vi "getSciScan image reference.vi"(8 "Error In":errorcluster, 11 "Image Refnum (Generic)":refnum<vi>) -> (0 "Error Out":errorcluster, 1 "Channel Number":u32, 2 "SciScan Image Tab Number":u32, 3 "Current Image":T1, 4 "Channel type":string)   [LabVIEW 2012]
doc: "SciScan 1.2 160622\nThis SubVI is part of the position control module.\nIts functionality is to manage the UI components related to display of images (in both the top level GUI and the position save UI)"
uses:
  <vilib>/vision/Image Controls.llb/IMAQ Image.ctl
  Custom Controls/display palette control.ctl
  GFG/GFGImageRefsGet.vi
  GFG/GFGfpRefGet.vi
  GFG/GFG library.lvlib
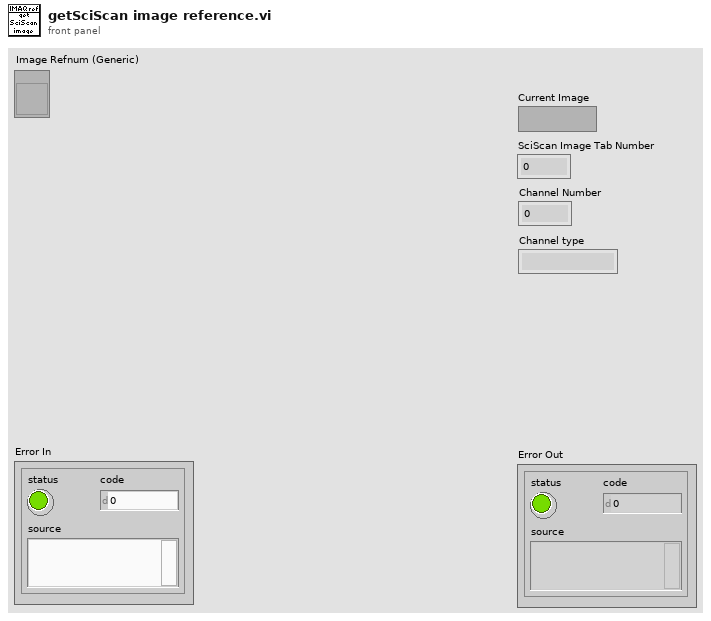
[diagram p1: front panel]
types:
  T1 = typedef "IMAQ Image.ctl" = refnum<image>
  T2 = typedef "display palette control.ctl" = enum16{"standard", "high clipping red", "low clipping blue", "high and low clipping", "high / low (full range)"}
  T3 = cluster{"Channel 1 small":T1, "Channel 2 small":T1, "Channel 3 small":T1, "Channel 4 small":T1, "Channel 1 large":T1, "Channel 2 large":T1, "Channel 3 large":T1, "Channel 4 large":T1, "RGB overlay":T1, "ROI Image display":T1, "arb line scan display":T1, "Channel 5 large":T1}
  T4 = cluster{"WaveformChartRef":refnum<vi>, "DigitalRef":refnum<vi>, "ArrayRef":refnum<vi>, "TabControlRef":refnum<vi>, "EnumRef":refnum<vi>, "RingRef":refnum<vi>, "BooleanRef":refnum<vi>, "KnobRef":refnum<vi>, "SlideRef":refnum<vi>, "PathRef":refnum<vi>, "StringRef":refnum<vi>, "ComboBox":refnum<vi>, "WaveformGraphRef":refnum<vi>}
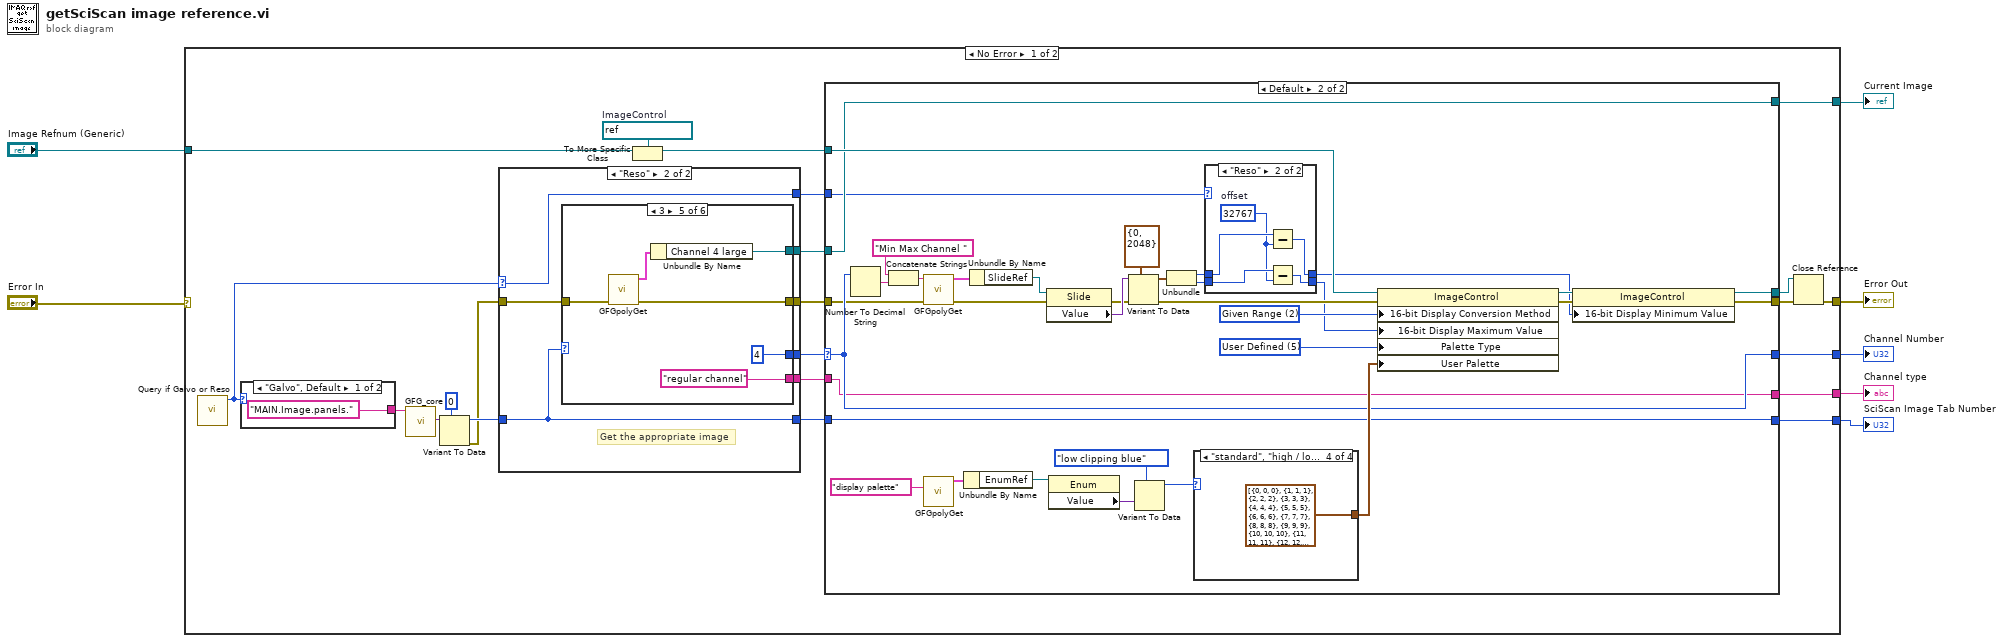
[diagram p0: block diagram]
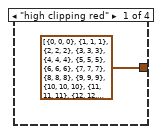
[diagram p4: hidden frame]
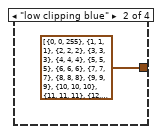
[diagram p5: hidden frame]
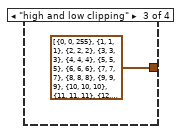
[diagram p6: hidden frame]
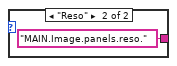
[diagram p7: hidden frame]
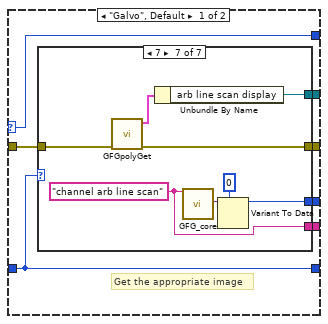
[diagram p8: hidden frame]
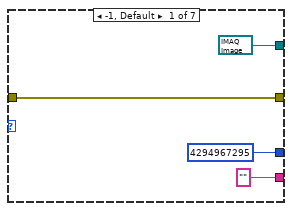
[diagram p9: hidden frame]
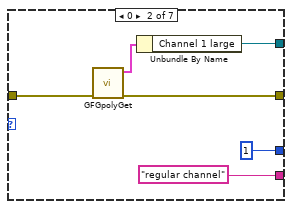
[diagram p10: hidden frame]
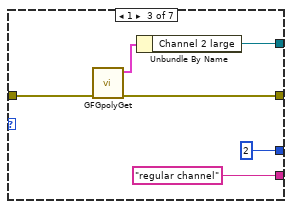
[diagram p11: hidden frame]
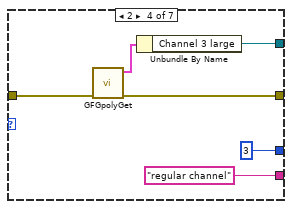
[diagram p12: hidden frame]
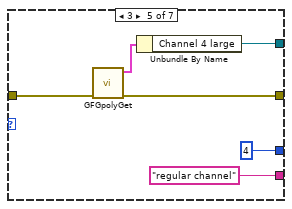
[diagram p13: hidden frame]
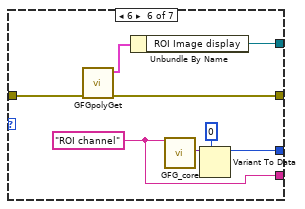
[diagram p14: hidden frame]
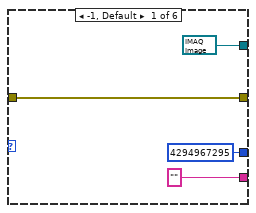
[diagram p15: hidden frame]
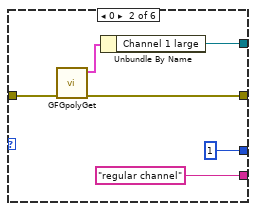
[diagram p16: hidden frame]
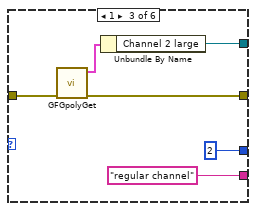
[diagram p17: hidden frame]
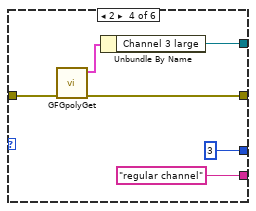
[diagram p18: hidden frame]
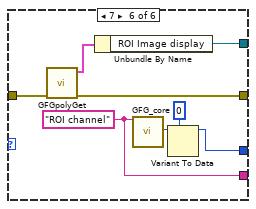
[diagram p19: hidden frame]
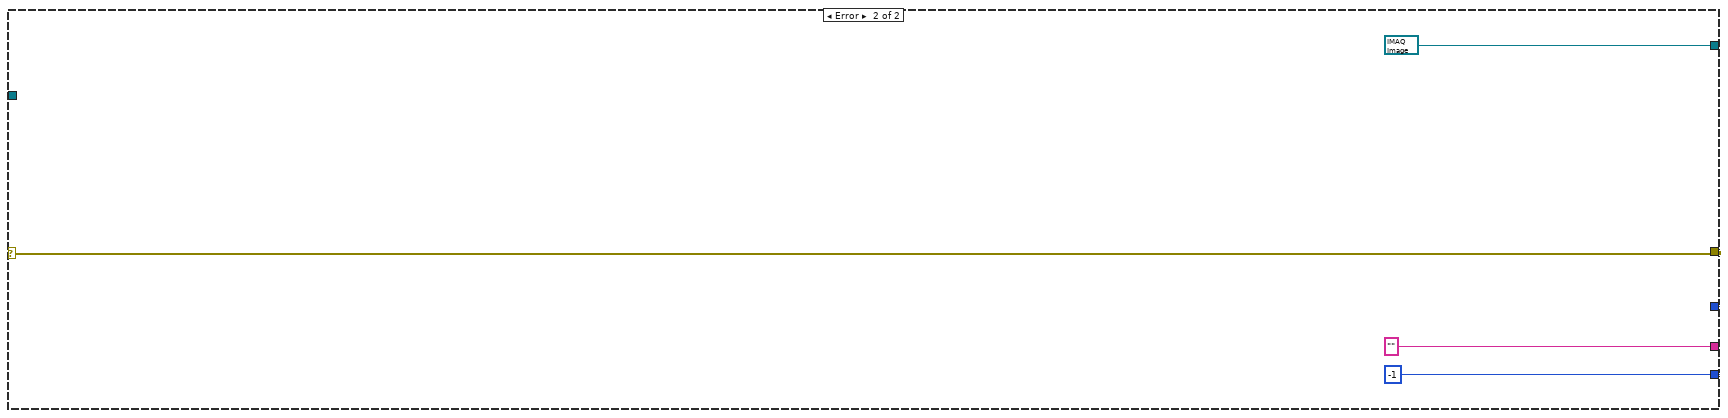
[diagram p20: hidden frame]
diagram:
  n1 = case shown="No Error" "Error In" {
    selector: "Error In" -> [_ w181]
    tunnel: "Image Refnum (Generic)" -> [w17 _]
    tunnel: [w22 w181] -> w5
    tunnel: [w14 T1 refnum ("Channel 4 large")] -> w4
    tunnel: [w11 w179] -> w3
    tunnel: [w13 w179] -> w2
    tunnel: [w9 "" ("Variable Name in")] -> w1
    frame No Error {
      w18 = refnum<vi> refnum  # ImageControl
      n2 = call "Query if Galvo or Reso.vi"() -> ("System Type"=w24:enum16{"Galvo", "Reso"})  [unwired: 10 in, 1 out]
      n3 = case shown="\"Galvo\", Default" w24 {
        tunnel: ["MAIN.Image.panels." ("Variable Name in") "MAIN.Image.panels.reso." ("Variable Name in")] -> w27
        frame "Galvo", Default {
        }
        frame "Reso" {
        }
      }
      n4 = call "GFG_core.vi"("Variable Name in"=w27) -> ("Variant Out"=w25:variant)  [unwired: 12 in, 6 out]
      n5 = Variant To Data(type=u32 0, Variant=w25) -> (data=w23:u32, error out=w21:errorcluster)  [unwired: 1 in]
      n6 = case shown="\"Reso\"" w24 {
        selector: w24 -> [w84 w135]
        tunnel: w21 -> [w90 w141]
        tunnel: w23 -> [w87 w138]
        tunnel: [w89 w140] -> w19
        tunnel: [w88 w139] -> w15
        tunnel: [w87 w138] -> w12
        tunnel: [w86 w137] -> w20
        tunnel: [w85 w136] -> w10
        tunnel: [w84 w135] -> w8
        frame "Galvo", Default {
          # "Get the appropriate image"
          n7 = case shown="7" w87 {
            tunnel: w90 -> [w93 w99 w105 w111 w117 w125 w133]
            tunnel: [w93 w98 w104 w110 w116 w124 w132] -> w89
            tunnel: [T1 refnum ("Channel 4 large") w97 w103 w109 w115 w123 w131] -> w88
            tunnel: [u32 4294967295 u32 1 u32 2 u32 3 u32 4 w120 w128] -> w86
            tunnel: ["" ("Variable Name in") "regular channel" ("Variable Name in") "regular channel" ("Variable Name in") "regular channel" ("Variable Name in") "regular channel" ("Variable Name in") w119 w127] -> w85
            frame -1, Default {
            }
            frame 0 {
              n8 = call-poly "GFGpolyGet.vi"("error in (no error)"=w99) -> ("error out"=w98:errorcluster, "Image Refs Out"=w100:T3)  [unwired: 9 in]
              n9 = Unbundle By Name(w100) -> ("Channel 1 large"=w97:T1)
            }
            frame 1 {
              n10 = call-poly "GFGpolyGet.vi"("error in (no error)"=w105) -> ("error out"=w104:errorcluster, "Image Refs Out"=w106:T3)  [unwired: 9 in]
              n11 = Unbundle By Name(w106) -> ("Channel 2 large"=w103:T1)
            }
            frame 2 {
              n12 = call-poly "GFGpolyGet.vi"("error in (no error)"=w111) -> ("error out"=w110:errorcluster, "Image Refs Out"=w112:T3)  [unwired: 9 in]
              n13 = Unbundle By Name(w112) -> ("Channel 3 large"=w109:T1)
            }
            frame 3 {
              n14 = call-poly "GFGpolyGet.vi"("error in (no error)"=w117) -> ("error out"=w116:errorcluster, "Image Refs Out"=w118:T3)  [unwired: 9 in]
              n15 = Unbundle By Name(w118) -> ("Channel 4 large"=w115:T1)
            }
            frame 6 {
              w119 = "ROI channel" ("Variable Name in")
              n16 = call-poly "GFGpolyGet.vi"("error in (no error)"=w125) -> ("error out"=w124:errorcluster, "Image Refs Out"=w126:T3)  [unwired: 9 in]
              n17 = Unbundle By Name(w126) -> ("ROI Image display"=w123:T1)
              n18 = call "GFG_core.vi"("Variable Name in"=w119) -> ("Variant Out"=w121:variant)  [unwired: 12 in, 6 out]
              n19 = Variant To Data(type=u32 0, Variant=w121) -> (data=w120:u32)  [unwired: 1 in, 1 out]
            }
            frame 7 {
              w127 = "channel arb line scan" ("Variable Name in")
              n20 = call-poly "GFGpolyGet.vi"("error in (no error)"=w133) -> ("error out"=w132:errorcluster, "Image Refs Out"=w134:T3)  [unwired: 9 in]
              n21 = Unbundle By Name(w134) -> ("arb line scan display"=w131:T1)
              n22 = call "GFG_core.vi"("Variable Name in"=w127) -> ("Variant Out"=w129:variant)  [unwired: 12 in, 6 out]
              n23 = Variant To Data(type=u32 0, Variant=w129) -> (data=w128:u32)  [unwired: 1 in, 1 out]
            }
          }
        }
        frame "Reso" {
          # "Get the appropriate image"
          n24 = case shown="3" w138 {
            tunnel: w141 -> [w144 w150 w156 w162 w168 w176]
            tunnel: [w144 w149 w155 w161 w167 w175] -> w140
            tunnel: [T1 refnum ("Channel 4 large") w148 w154 w160 w166 w174] -> w139
            tunnel: [u32 4294967295 u32 1 u32 2 u32 3 u32 4 w171] -> w137
            tunnel: ["" ("Variable Name in") "regular channel" ("Variable Name in") "regular channel" ("Variable Name in") "regular channel" ("Variable Name in") "regular channel" ("Variable Name in") w170] -> w136
            frame -1, Default {
            }
            frame 0 {
              n25 = call-poly "GFGpolyGet.vi"("error in (no error)"=w150) -> ("error out"=w149:errorcluster, "Image Refs Out"=w151:T3)  [unwired: 9 in]
              n26 = Unbundle By Name(w151) -> ("Channel 1 large"=w148:T1)
            }
            frame 1 {
              n27 = call-poly "GFGpolyGet.vi"("error in (no error)"=w156) -> ("error out"=w155:errorcluster, "Image Refs Out"=w157:T3)  [unwired: 9 in]
              n28 = Unbundle By Name(w157) -> ("Channel 2 large"=w154:T1)
            }
            frame 2 {
              n29 = call-poly "GFGpolyGet.vi"("error in (no error)"=w162) -> ("error out"=w161:errorcluster, "Image Refs Out"=w163:T3)  [unwired: 9 in]
              n30 = Unbundle By Name(w163) -> ("Channel 3 large"=w160:T1)
            }
            frame 3 {
              n31 = call-poly "GFGpolyGet.vi"("error in (no error)"=w168) -> ("error out"=w167:errorcluster, "Image Refs Out"=w169:T3)  [unwired: 9 in]
              n32 = Unbundle By Name(w169) -> ("Channel 4 large"=w166:T1)
            }
            frame 7 {
              w170 = "ROI channel" ("Variable Name in")
              n33 = call-poly "GFGpolyGet.vi"("error in (no error)"=w176) -> ("error out"=w175:errorcluster, "Image Refs Out"=w177:T3)  [unwired: 9 in]
              n34 = Unbundle By Name(w177) -> ("ROI Image display"=w174:T1)
              n35 = call "GFG_core.vi"("Variable Name in"=w170) -> ("Variant Out"=w172:variant)  [unwired: 12 in, 6 out]
              n36 = Variant To Data(type=u32 0, Variant=w172) -> (data=w171:u32)  [unwired: 1 in, 1 out]
            }
          }
        }
      }
      n37 = To More Specific Class(target class=w18, reference=w17) -> (specific class reference=w16:refnum<vi>)  [unwired: 1 in, 1 out]
      n38 = case shown="Default" w20 {
        selector: w20 -> [w32 w44]
        tunnel: w16 -> [w35 w46]
        tunnel: [w35 w48] -> w29
        tunnel: [w34 w47] -> w28
        tunnel: w19 -> [w34 w41]
        tunnel: w15 -> [w33 w45]
        tunnel: [w33 w45] -> w14
        tunnel: [w32 w44] -> w13
        tunnel: w12 -> [w31 w43]
        tunnel: [w31 w43] -> w11
        tunnel: w10 -> [w30 w42]
        tunnel: [w30 w42] -> w9
        tunnel: w8 -> [_ w40]
        frame 0, -1 {
        }
        frame Default {
          w52 = u32 5 items=["Grayscale", "Binary", "Gradient", "Rainbow", "Temperature", "User Defined"] ("Palette:Palette Type")
          w63 = u32 2 items=["Full Dynamic", "Downshift", "Given Range", "90% Dynamic", "Given Percent Range"] ("16-bit Display Mapping:Conversion Method")
          n39 = Number To Decimal String(number=w44) -> (decimal integer string=w66:string)  [unwired: 1 in]
          n40 = Concatenate Strings("Min Max Channel " ("Variable Name in"), w66) -> (w70:string)
          n41 = call-poly "GFGpolyGet.vi"("error in (no error)"=w41, "Variable Name in"=w70) -> ("error out"=w62:errorcluster, "output cluster"=w64:T4)  [unwired: 8 in]
          n42 = call-poly "GFGpolyGet.vi"("Variable Name in"="display palette") -> ("output cluster"=w56:T4)  [unwired: 9 in, 1 out]
          n43 = Unbundle By Name(w56) -> ("EnumRef"=w57:refnum<vi>)
          n44 = Unbundle By Name(w64) -> ("SlideRef"=w67:refnum<vi>)
          n45 = property class="Slide"(reference=w67, error in=w62) -> (error out=w61:errorcluster, "Value"=w68:variant)  [unwired: 1 out]
          n46 = property class="Enum"(reference=w57) -> ("Value"=w55:variant)  [unwired: 1 in, 2 out]
          n47 = Variant To Data(error in=w61, type=cluster{i32, i32} {0, 2048} ("channel1"), Variant=w68) -> (data=w59:cluster{i32, i32}, error out=w60:errorcluster)
          n48 = Variant To Data(type=display_palette_control."low clipping blue" ("display palette"), Variant=w55) -> (data=w53:T2)  [unwired: 1 in, 1 out]
          n49 = Unbundle(w59) -> (w39:i32, w38:i32)
          n50 = case shown="\"standard\", \"high / low (full range)\"" w53 {
            tunnel: [cluster{"Red":u8, "Green":u8, "Blue":u8}[] [{"Red"=0, "Green"=0, "Blue"=0}, {"Red"=1, "Green"=1, "Blue"=1}, {"Red"=2, "Green"=2, "Blue"=2}, {"Red"=3, "Green"=3, "Blue"=3}, {"Red"=4, "Green"=4, "Blue"=4}, {"Red"=5, "Green"=5, "Blue"=5}, {"Red"=6, "Green"=6, "Blue"=6}, {"Red"=7, "Green"=7, "Blue"=7}, {"Red"=8, "Green"=8, "Blue"=8}, {"Red"=9, "Green"=9, "Blue"=9}, {"Red"=10, "Green"=10, "Blue"=10}, {"Red"=11, "Green"=11, "Blue"=11}, {"Red"=12, "Green"=12, "Blue"=12}, {"Red"=13, "Green"=13, "Blue"=13}, {"Red"=14, "Green"=14, "Blue"=14}, {"Red"=15, "Green"=15, "Blue"=15}, {"Red"=16, "Green"=16, "Blue"=16}, {"Red"=17, "Green"=17, "Blue"=17}, {"Red"=18, "Green"=18, "Blue"=18}, {"Red"=19, "Green"=19, "Blue"=19}, {"Red"=20, "Green"=20, "Blue"=20}, {"Red"=21, "Green"=21, "Blue"=21}, {"Red"=22, "Green"=22, "Blue"=22}, {"Red"=23, "Green"=23, "Blue"=23}, {"Red"=24, "Green"=24, "Blue"=24}, {"Red"=25, "Green"=25, "Blue"=25}, {"Red"=26, "Green"=26, "Blue"=26}, {"Red"=27, "Green"=27, "Blue"=27}, {"Red"=28, "Green"=28, "Blue"=28}, {"Red"=29, "Green"=29, "Blue"=29}, {"Red"=30, "Green"=30, "Blue"=30}, {"Red"=31, "Green"=31, "Blue"=31}, {"Red"=32, "Green"=32, "Blue"=32}, {"Red"=33, "Green"=33, "Blue"=33}, {"Red"=34, "Green"=34, "Blue"=34}, {"Red"=35, "Green"=35, "Blue"=35}, {"Red"=36, "Green"=36, "Blue"=36}, {"Red"=37, "Green"=37, "Blue"=37}, {"Red"=38, "Green"=38, "Blue"=38}, {"Red"=39, "Green"=39, "Blue"=39}, {"Red"=40, "Green"=40, "Blue"=40}, {"Red"=41, "Green"=41, "Blue"=41}, {"Red"=42, "Green"=42, "Blue"=42}, {"Red"=43, "Green"=43, "Blue"=43}, {"Red"=44, "Green"=44, "Blue"=44}, {"Red"=45, "Green"=45, "Blue"=45}, {"Red"=46, "Green"=46, "Blue"=46}, {"Red"=47, "Green"=47, "Blue"=47}, {"Red"=48, "Green"=48, "Blue"=48}, {"Red"=49, "Green"=49, "Blue"=49}, {"Red"=50, "Green"=50, "Blue"=50}, {"Red"=51, "Green"=51, "Blue"=51}, {"Red"=52, "Green"=52, "Blue"=52}, {"Red"=53, "Green"=53, "Blue"=53}, {"Red"=54, "Green"=54, "Blue"=54}, {"Red"=55, "Green"=55, "Blue"=55}, {"Red"=56, "Green"=56, "Blue"=56}, {"Red"=57, "Green"=57, "Blue"=57}, {"Red"=58, "Green"=58, "Blue"=58}, {"Red"=59, "Green"=59, "Blue"=59}, {"Red"=60, "Green"=60, "Blue"=60}, {"Red"=61, "Green"=61, "Blue"=61}, {"Red"=62, "Green"=62, "Blue"=62}, {"Red"=63, "Green"=63, "Blue"=63}, {"Red"=64, "Green"=64, "Blue"=64}, {"Red"=65, "Green"=65, "Blue"=65}, {"Red"=66, "Green"=66, "Blue"=66}, {"Red"=67, "Green"=67, "Blue"=67}, {"Red"=68, "Green"=68, "Blue"=68}, {"Red"=69, "Green"=69, "Blue"=69}, {"Red"=70, "Green"=70, "Blue"=70}, {"Red"=71, "Green"=71, "Blue"=71}, {"Red"=72, "Green"=72, "Blue"=72}, {"Red"=73, "Green"=73, "Blue"=73}, {"Red"=74, "Green"=74, "Blue"=74}, {"Red"=75, "Green"=75, "Blue"=75}, {"Red"=76, "Green"=76, "Blue"=76}, {"Red"=77, "Green"=77, "Blue"=77}, {"Red"=78, "Green"=78, "Blue"=78}, {"Red"=79, "Green"=79, "Blue"=79}, {"Red"=80, "Green"=80, "Blue"=80}, {"Red"=81, "Green"=81, "Blue"=81}, {"Red"=82, "Green"=82, "Blue"=82}, {"Red"=83, "Green"=83, "Blue"=83}, {"Red"=84, "Green"=84, "Blue"=84}, {"Red"=85, "Green"=85, "Blue"=85}, {"Red"=86, "Green"=86, "Blue"=86}, {"Red"=87, "Green"=87, "Blue"=87}, {"Red"=88, "Green"=88, "Blue"=88}, {"Red"=89, "Green"=89, "Blue"=89}, {"Red"=90, "Green"=90, "Blue"=90}, {"Red"=91, "Green"=91, "Blue"=91}, {"Red"=92, "Green"=92, "Blue"=92}, {"Red"=93, "Green"=93, "Blue"=93}, {"Red"=94, "Green"=94, "Blue"=94}, {"Red"=95, "Green"=95, "Blue"=95}, {"Red"=96, "Green"=96, "Blue"=96}, {"Red"=97, "Green"=97, "Blue"=97}, {"Red"=98, "Green"=98, "Blue"=98}, {"Red"=99, "Green"=99, "Blue"=99}, {"Red"=100, "Green"=100, "Blue"=100}, {"Red"=101, "Green"=101, "Blue"=101}, {"Red"=102, "Green"=102, "Blue"=102}, {"Red"=103, "Green"=103, "Blue"=103}, {"Red"=104, "Green"=104, "Blue"=104}, {"Red"=105, "Green"=105, "Blue"=105}, {"Red"=106, "Green"=106, "Blue"=106}, {"Red"=107, "Green"=107, "Blue"=107}, {"Red"=108, "Green"=108, "Blue"=108}, {"Red"=109, "Green"=109, "Blue"=109}, {"Red"=110, "Green"=110, "Blue"=110}, {"Red"=111, "Green"=111, "Blue"=111}, {"Red"=112, "Green"=112, "Blue"=112}, {"Red"=113, "Green"=113, "Blue"=113}, {"Red"=114, "Green"=114, "Blue"=114}, {"Red"=115, "Green"=115, "Blue"=115}, {"Red"=116, "Green"=116, "Blue"=116}, {"Red"=117, "Green"=117, "Blue"=117}, {"Red"=118, "Green"=118, "Blue"=118}, {"Red"=119, "Green"=119, "Blue"=119}, {"Red"=120, "Green"=120, "Blue"=120}, {"Red"=121, "Green"=121, "Blue"=121}, {"Red"=122, "Green"=122, "Blue"=122}, {"Red"=123, "Green"=123, "Blue"=123}, {"Red"=124, "Green"=124, "Blue"=124}, {"Red"=125, "Green"=125, "Blue"=125}, {"Red"=126, "Green"=126, "Blue"=126}, {"Red"=127, "Green"=127, "Blue"=127}, {"Red"=128, "Green"=128, "Blue"=128}, {"Red"=129, "Green"=129, "Blue"=129}, {"Red"=130, "Green"=130, "Blue"=130}, {"Red"=131, "Green"=131, "Blue"=131}, {"Red"=132, "Green"=132, "Blue"=132}, {"Red"=133, "Green"=133, "Blue"=133}, {"Red"=134, "Green"=134, "Blue"=134}, {"Red"=135, "Green"=135, "Blue"=135}, {"Red"=136, "Green"=136, "Blue"=136}, {"Red"=137, "Green"=137, "Blue"=137}, {"Red"=138, "Green"=138, "Blue"=138}, {"Red"=139, "Green"=139, "Blue"=139}, {"Red"=140, "Green"=140, "Blue"=140}, {"Red"=141, "Green"=141, "Blue"=141}, {"Red"=142, "Green"=142, "Blue"=142}, {"Red"=143, "Green"=143, "Blue"=143}, {"Red"=144, "Green"=144, "Blue"=144}, {"Red"=145, "Green"=145, "Blue"=145}, {"Red"=146, "Green"=146, "Blue"=146}, {"Red"=147, "Green"=147, "Blue"=147}, {"Red"=148, "Green"=148, "Blue"=148}, {"Red"=149, "Green"=149, "Blue"=149}, {"Red"=150, "Green"=150, "Blue"=150}, {"Red"=151, "Green"=151, "Blue"=151}, {"Red"=152, "Green"=152, "Blue"=152}, {"Red"=153, "Green"=153, "Blue"=153}, {"Red"=154, "Green"=154, "Blue"=154}, {"Red"=155, "Green"=155, "Blue"=155}, {"Red"=156, "Green"=156, "Blue"=156}, {"Red"=157, "Green"=157, "Blue"=157}, {"Red"=158, "Green"=158, "Blue"=158}, {"Red"=159, "Green"=159, "Blue"=159}, {"Red"=160, "Green"=160, "Blue"=160}, {"Red"=161, "Green"=161, "Blue"=161}, {"Red"=162, "Green"=162, "Blue"=162}, {"Red"=163, "Green"=163, "Blue"=163}, {"Red"=164, "Green"=164, "Blue"=164}, {"Red"=165, "Green"=165, "Blue"=165}, {"Red"=166, "Green"=166, "Blue"=166}, {"Red"=167, "Green"=167, "Blue"=167}, {"Red"=168, "Green"=168, "Blue"=168}, {"Red"=169, "Green"=169, "Blue"=169}, {"Red"=170, "Green"=170, "Blue"=170}, {"Red"=171, "Green"=171, "Blue"=171}, {"Red"=172, "Green"=172, "Blue"=172}, {"Red"=173, "Green"=173, "Blue"=173}, {"Red"=174, "Green"=174, "Blue"=174}, {"Red"=175, "Green"=175, "Blue"=175}, {"Red"=176, "Green"=176, "Blue"=176}, {"Red"=177, "Green"=177, "Blue"=177}, {"Red"=178, "Green"=178, "Blue"=178}, {"Red"=179, "Green"=179, "Blue"=179}, {"Red"=180, "Green"=180, "Blue"=180}, {"Red"=181, "Green"=181, "Blue"=181}, {"Red"=182, "Green"=182, "Blue"=182}, {"Red"=183, "Green"=183, "Blue"=183}, {"Red"=184, "Green"=184, "Blue"=184}, {"Red"=185, "Green"=185, "Blue"=185}, {"Red"=186, "Green"=186, "Blue"=186}, {"Red"=187, "Green"=187, "Blue"=187}, {"Red"=188, "Green"=188, "Blue"=188}, {"Red"=189, "Green"=189, "Blue"=189}, {"Red"=190, "Green"=190, "Blue"=190}, {"Red"=191, "Green"=191, "Blue"=191}, {"Red"=192, "Green"=192, "Blue"=192}, {"Red"=193, "Green"=193, "Blue"=193}, {"Red"=194, "Green"=194, "Blue"=194}, {"Red"=195, "Green"=195, "Blue"=195}, {"Red"=196, "Green"=196, "Blue"=196}, {"Red"=197, "Green"=197, "Blue"=197}, {"Red"=198, "Green"=198, "Blue"=198}, {"Red"=199, "Green"=199, "Blue"=199}, {"Red"=200, "Green"=200, "Blue"=200}, {"Red"=201, "Green"=201, "Blue"=201}, {"Red"=202, "Green"=202, "Blue"=202}, {"Red"=203, "Green"=203, "Blue"=203}, {"Red"=204, "Green"=204, "Blue"=204}, {"Red"=205, "Green"=205, "Blue"=205}, {"Red"=206, "Green"=206, "Blue"=206}, {"Red"=207, "Green"=207, "Blue"=207}, {"Red"=208, "Green"=208, "Blue"=208}, {"Red"=209, "Green"=209, "Blue"=209}, {"Red"=210, "Green"=210, "Blue"=210}, {"Red"=211, "Green"=211, "Blue"=211}, {"Red"=212, "Green"=212, "Blue"=212}, {"Red"=213, "Green"=213, "Blue"=213}, {"Red"=214, "Green"=214, "Blue"=214}, {"Red"=215, "Green"=215, "Blue"=215}, {"Red"=216, "Green"=216, "Blue"=216}, {"Red"=217, "Green"=217, "Blue"=217}, {"Red"=218, "Green"=218, "Blue"=218}, {"Red"=219, "Green"=219, "Blue"=219}, {"Red"=220, "Green"=220, "Blue"=220}, {"Red"=221, "Green"=221, "Blue"=221}, {"Red"=222, "Green"=222, "Blue"=222}, {"Red"=223, "Green"=223, "Blue"=223}, {"Red"=224, "Green"=224, "Blue"=224}, {"Red"=225, "Green"=225, "Blue"=225}, {"Red"=226, "Green"=226, "Blue"=226}, {"Red"=227, "Green"=227, "Blue"=227}, {"Red"=228, "Green"=228, "Blue"=228}, {"Red"=229, "Green"=229, "Blue"=229}, {"Red"=230, "Green"=230, "Blue"=230}, {"Red"=231, "Green"=231, "Blue"=231}, {"Red"=232, "Green"=232, "Blue"=232}, {"Red"=233, "Green"=233, "Blue"=233}, {"Red"=234, "Green"=234, "Blue"=234}, {"Red"=235, "Green"=235, "Blue"=235}, {"Red"=236, "Green"=236, "Blue"=236}, {"Red"=237, "Green"=237, "Blue"=237}, {"Red"=238, "Green"=238, "Blue"=238}, {"Red"=239, "Green"=239, "Blue"=239}, {"Red"=240, "Green"=240, "Blue"=240}, {"Red"=241, "Green"=241, "Blue"=241}, {"Red"=242, "Green"=242, "Blue"=242}, {"Red"=243, "Green"=243, "Blue"=243}, {"Red"=244, "Green"=244, "Blue"=244}, {"Red"=245, "Green"=245, "Blue"=245}, {"Red"=246, "Green"=246, "Blue"=246}, {"Red"=247, "Green"=247, "Blue"=247}, {"Red"=248, "Green"=248, "Blue"=248}, {"Red"=249, "Green"=249, "Blue"=249}, {"Red"=250, "Green"=250, "Blue"=250}, {"Red"=251, "Green"=251, "Blue"=251}, {"Red"=252, "Green"=252, "Blue"=252}, {"Red"=253, "Green"=253, "Blue"=253}, {"Red"=254, "Green"=254, "Blue"=254}, {"Red"=255, "Green"=0, "Blue"=0}] ("Color Palette") cluster{"Red":u8, "Green":u8, "Blue":u8}[] [{"Red"=0, "Green"=0, "Blue"=255}, {"Red"=1, "Green"=1, "Blue"=1}, {"Red"=2, "Green"=2, "Blue"=2}, {"Red"=3, "Green"=3, "Blue"=3}, {"Red"=4, "Green"=4, "Blue"=4}, {"Red"=5, "Green"=5, "Blue"=5}, {"Red"=6, "Green"=6, "Blue"=6}, {"Red"=7, "Green"=7, "Blue"=7}, {"Red"=8, "Green"=8, "Blue"=8}, {"Red"=9, "Green"=9, "Blue"=9}, {"Red"=10, "Green"=10, "Blue"=10}, {"Red"=11, "Green"=11, "Blue"=11}, {"Red"=12, "Green"=12, "Blue"=12}, {"Red"=13, "Green"=13, "Blue"=13}, {"Red"=14, "Green"=14, "Blue"=14}, {"Red"=15, "Green"=15, "Blue"=15}, {"Red"=16, "Green"=16, "Blue"=16}, {"Red"=17, "Green"=17, "Blue"=17}, {"Red"=18, "Green"=18, "Blue"=18}, {"Red"=19, "Green"=19, "Blue"=19}, {"Red"=20, "Green"=20, "Blue"=20}, {"Red"=21, "Green"=21, "Blue"=21}, {"Red"=22, "Green"=22, "Blue"=22}, {"Red"=23, "Green"=23, "Blue"=23}, {"Red"=24, "Green"=24, "Blue"=24}, {"Red"=25, "Green"=25, "Blue"=25}, {"Red"=26, "Green"=26, "Blue"=26}, {"Red"=27, "Green"=27, "Blue"=27}, {"Red"=28, "Green"=28, "Blue"=28}, {"Red"=29, "Green"=29, "Blue"=29}, {"Red"=30, "Green"=30, "Blue"=30}, {"Red"=31, "Green"=31, "Blue"=31}, {"Red"=32, "Green"=32, "Blue"=32}, {"Red"=33, "Green"=33, "Blue"=33}, {"Red"=34, "Green"=34, "Blue"=34}, {"Red"=35, "Green"=35, "Blue"=35}, {"Red"=36, "Green"=36, "Blue"=36}, {"Red"=37, "Green"=37, "Blue"=37}, {"Red"=38, "Green"=38, "Blue"=38}, {"Red"=39, "Green"=39, "Blue"=39}, {"Red"=40, "Green"=40, "Blue"=40}, {"Red"=41, "Green"=41, "Blue"=41}, {"Red"=42, "Green"=42, "Blue"=42}, {"Red"=43, "Green"=43, "Blue"=43}, {"Red"=44, "Green"=44, "Blue"=44}, {"Red"=45, "Green"=45, "Blue"=45}, {"Red"=46, "Green"=46, "Blue"=46}, {"Red"=47, "Green"=47, "Blue"=47}, {"Red"=48, "Green"=48, "Blue"=48}, {"Red"=49, "Green"=49, "Blue"=49}, {"Red"=50, "Green"=50, "Blue"=50}, {"Red"=51, "Green"=51, "Blue"=51}, {"Red"=52, "Green"=52, "Blue"=52}, {"Red"=53, "Green"=53, "Blue"=53}, {"Red"=54, "Green"=54, "Blue"=54}, {"Red"=55, "Green"=55, "Blue"=55}, {"Red"=56, "Green"=56, "Blue"=56}, {"Red"=57, "Green"=57, "Blue"=57}, {"Red"=58, "Green"=58, "Blue"=58}, {"Red"=59, "Green"=59, "Blue"=59}, {"Red"=60, "Green"=60, "Blue"=60}, {"Red"=61, "Green"=61, "Blue"=61}, {"Red"=62, "Green"=62, "Blue"=62}, {"Red"=63, "Green"=63, "Blue"=63}, {"Red"=64, "Green"=64, "Blue"=64}, {"Red"=65, "Green"=65, "Blue"=65}, {"Red"=66, "Green"=66, "Blue"=66}, {"Red"=67, "Green"=67, "Blue"=67}, {"Red"=68, "Green"=68, "Blue"=68}, {"Red"=69, "Green"=69, "Blue"=69}, {"Red"=70, "Green"=70, "Blue"=70}, {"Red"=71, "Green"=71, "Blue"=71}, {"Red"=72, "Green"=72, "Blue"=72}, {"Red"=73, "Green"=73, "Blue"=73}, {"Red"=74, "Green"=74, "Blue"=74}, {"Red"=75, "Green"=75, "Blue"=75}, {"Red"=76, "Green"=76, "Blue"=76}, {"Red"=77, "Green"=77, "Blue"=77}, {"Red"=78, "Green"=78, "Blue"=78}, {"Red"=79, "Green"=79, "Blue"=79}, {"Red"=80, "Green"=80, "Blue"=80}, {"Red"=81, "Green"=81, "Blue"=81}, {"Red"=82, "Green"=82, "Blue"=82}, {"Red"=83, "Green"=83, "Blue"=83}, {"Red"=84, "Green"=84, "Blue"=84}, {"Red"=85, "Green"=85, "Blue"=85}, {"Red"=86, "Green"=86, "Blue"=86}, {"Red"=87, "Green"=87, "Blue"=87}, {"Red"=88, "Green"=88, "Blue"=88}, {"Red"=89, "Green"=89, "Blue"=89}, {"Red"=90, "Green"=90, "Blue"=90}, {"Red"=91, "Green"=91, "Blue"=91}, {"Red"=92, "Green"=92, "Blue"=92}, {"Red"=93, "Green"=93, "Blue"=93}, {"Red"=94, "Green"=94, "Blue"=94}, {"Red"=95, "Green"=95, "Blue"=95}, {"Red"=96, "Green"=96, "Blue"=96}, {"Red"=97, "Green"=97, "Blue"=97}, {"Red"=98, "Green"=98, "Blue"=98}, {"Red"=99, "Green"=99, "Blue"=99}, {"Red"=100, "Green"=100, "Blue"=100}, {"Red"=101, "Green"=101, "Blue"=101}, {"Red"=102, "Green"=102, "Blue"=102}, {"Red"=103, "Green"=103, "Blue"=103}, {"Red"=104, "Green"=104, "Blue"=104}, {"Red"=105, "Green"=105, "Blue"=105}, {"Red"=106, "Green"=106, "Blue"=106}, {"Red"=107, "Green"=107, "Blue"=107}, {"Red"=108, "Green"=108, "Blue"=108}, {"Red"=109, "Green"=109, "Blue"=109}, {"Red"=110, "Green"=110, "Blue"=110}, {"Red"=111, "Green"=111, "Blue"=111}, {"Red"=112, "Green"=112, "Blue"=112}, {"Red"=113, "Green"=113, "Blue"=113}, {"Red"=114, "Green"=114, "Blue"=114}, {"Red"=115, "Green"=115, "Blue"=115}, {"Red"=116, "Green"=116, "Blue"=116}, {"Red"=117, "Green"=117, "Blue"=117}, {"Red"=118, "Green"=118, "Blue"=118}, {"Red"=119, "Green"=119, "Blue"=119}, {"Red"=120, "Green"=120, "Blue"=120}, {"Red"=121, "Green"=121, "Blue"=121}, {"Red"=122, "Green"=122, "Blue"=122}, {"Red"=123, "Green"=123, "Blue"=123}, {"Red"=124, "Green"=124, "Blue"=124}, {"Red"=125, "Green"=125, "Blue"=125}, {"Red"=126, "Green"=126, "Blue"=126}, {"Red"=127, "Green"=127, "Blue"=127}, {"Red"=128, "Green"=128, "Blue"=128}, {"Red"=129, "Green"=129, "Blue"=129}, {"Red"=130, "Green"=130, "Blue"=130}, {"Red"=131, "Green"=131, "Blue"=131}, {"Red"=132, "Green"=132, "Blue"=132}, {"Red"=133, "Green"=133, "Blue"=133}, {"Red"=134, "Green"=134, "Blue"=134}, {"Red"=135, "Green"=135, "Blue"=135}, {"Red"=136, "Green"=136, "Blue"=136}, {"Red"=137, "Green"=137, "Blue"=137}, {"Red"=138, "Green"=138, "Blue"=138}, {"Red"=139, "Green"=139, "Blue"=139}, {"Red"=140, "Green"=140, "Blue"=140}, {"Red"=141, "Green"=141, "Blue"=141}, {"Red"=142, "Green"=142, "Blue"=142}, {"Red"=143, "Green"=143, "Blue"=143}, {"Red"=144, "Green"=144, "Blue"=144}, {"Red"=145, "Green"=145, "Blue"=145}, {"Red"=146, "Green"=146, "Blue"=146}, {"Red"=147, "Green"=147, "Blue"=147}, {"Red"=148, "Green"=148, "Blue"=148}, {"Red"=149, "Green"=149, "Blue"=149}, {"Red"=150, "Green"=150, "Blue"=150}, {"Red"=151, "Green"=151, "Blue"=151}, {"Red"=152, "Green"=152, "Blue"=152}, {"Red"=153, "Green"=153, "Blue"=153}, {"Red"=154, "Green"=154, "Blue"=154}, {"Red"=155, "Green"=155, "Blue"=155}, {"Red"=156, "Green"=156, "Blue"=156}, {"Red"=157, "Green"=157, "Blue"=157}, {"Red"=158, "Green"=158, "Blue"=158}, {"Red"=159, "Green"=159, "Blue"=159}, {"Red"=160, "Green"=160, "Blue"=160}, {"Red"=161, "Green"=161, "Blue"=161}, {"Red"=162, "Green"=162, "Blue"=162}, {"Red"=163, "Green"=163, "Blue"=163}, {"Red"=164, "Green"=164, "Blue"=164}, {"Red"=165, "Green"=165, "Blue"=165}, {"Red"=166, "Green"=166, "Blue"=166}, {"Red"=167, "Green"=167, "Blue"=167}, {"Red"=168, "Green"=168, "Blue"=168}, {"Red"=169, "Green"=169, "Blue"=169}, {"Red"=170, "Green"=170, "Blue"=170}, {"Red"=171, "Green"=171, "Blue"=171}, {"Red"=172, "Green"=172, "Blue"=172}, {"Red"=173, "Green"=173, "Blue"=173}, {"Red"=174, "Green"=174, "Blue"=174}, {"Red"=175, "Green"=175, "Blue"=175}, {"Red"=176, "Green"=176, "Blue"=176}, {"Red"=177, "Green"=177, "Blue"=177}, {"Red"=178, "Green"=178, "Blue"=178}, {"Red"=179, "Green"=179, "Blue"=179}, {"Red"=180, "Green"=180, "Blue"=180}, {"Red"=181, "Green"=181, "Blue"=181}, {"Red"=182, "Green"=182, "Blue"=182}, {"Red"=183, "Green"=183, "Blue"=183}, {"Red"=184, "Green"=184, "Blue"=184}, {"Red"=185, "Green"=185, "Blue"=185}, {"Red"=186, "Green"=186, "Blue"=186}, {"Red"=187, "Green"=187, "Blue"=187}, {"Red"=188, "Green"=188, "Blue"=188}, {"Red"=189, "Green"=189, "Blue"=189}, {"Red"=190, "Green"=190, "Blue"=190}, {"Red"=191, "Green"=191, "Blue"=191}, {"Red"=192, "Green"=192, "Blue"=192}, {"Red"=193, "Green"=193, "Blue"=193}, {"Red"=194, "Green"=194, "Blue"=194}, {"Red"=195, "Green"=195, "Blue"=195}, {"Red"=196, "Green"=196, "Blue"=196}, {"Red"=197, "Green"=197, "Blue"=197}, {"Red"=198, "Green"=198, "Blue"=198}, {"Red"=199, "Green"=199, "Blue"=199}, {"Red"=200, "Green"=200, "Blue"=200}, {"Red"=201, "Green"=201, "Blue"=201}, {"Red"=202, "Green"=202, "Blue"=202}, {"Red"=203, "Green"=203, "Blue"=203}, {"Red"=204, "Green"=204, "Blue"=204}, {"Red"=205, "Green"=205, "Blue"=205}, {"Red"=206, "Green"=206, "Blue"=206}, {"Red"=207, "Green"=207, "Blue"=207}, {"Red"=208, "Green"=208, "Blue"=208}, {"Red"=209, "Green"=209, "Blue"=209}, {"Red"=210, "Green"=210, "Blue"=210}, {"Red"=211, "Green"=211, "Blue"=211}, {"Red"=212, "Green"=212, "Blue"=212}, {"Red"=213, "Green"=213, "Blue"=213}, {"Red"=214, "Green"=214, "Blue"=214}, {"Red"=215, "Green"=215, "Blue"=215}, {"Red"=216, "Green"=216, "Blue"=216}, {"Red"=217, "Green"=217, "Blue"=217}, {"Red"=218, "Green"=218, "Blue"=218}, {"Red"=219, "Green"=219, "Blue"=219}, {"Red"=220, "Green"=220, "Blue"=220}, {"Red"=221, "Green"=221, "Blue"=221}, {"Red"=222, "Green"=222, "Blue"=222}, {"Red"=223, "Green"=223, "Blue"=223}, {"Red"=224, "Green"=224, "Blue"=224}, {"Red"=225, "Green"=225, "Blue"=225}, {"Red"=226, "Green"=226, "Blue"=226}, {"Red"=227, "Green"=227, "Blue"=227}, {"Red"=228, "Green"=228, "Blue"=228}, {"Red"=229, "Green"=229, "Blue"=229}, {"Red"=230, "Green"=230, "Blue"=230}, {"Red"=231, "Green"=231, "Blue"=231}, {"Red"=232, "Green"=232, "Blue"=232}, {"Red"=233, "Green"=233, "Blue"=233}, {"Red"=234, "Green"=234, "Blue"=234}, {"Red"=235, "Green"=235, "Blue"=235}, {"Red"=236, "Green"=236, "Blue"=236}, {"Red"=237, "Green"=237, "Blue"=237}, {"Red"=238, "Green"=238, "Blue"=238}, {"Red"=239, "Green"=239, "Blue"=239}, {"Red"=240, "Green"=240, "Blue"=240}, {"Red"=241, "Green"=241, "Blue"=241}, {"Red"=242, "Green"=242, "Blue"=242}, {"Red"=243, "Green"=243, "Blue"=243}, {"Red"=244, "Green"=244, "Blue"=244}, {"Red"=245, "Green"=245, "Blue"=245}, {"Red"=246, "Green"=246, "Blue"=246}, {"Red"=247, "Green"=247, "Blue"=247}, {"Red"=248, "Green"=248, "Blue"=248}, {"Red"=249, "Green"=249, "Blue"=249}, {"Red"=250, "Green"=250, "Blue"=250}, {"Red"=251, "Green"=251, "Blue"=251}, {"Red"=252, "Green"=252, "Blue"=252}, {"Red"=253, "Green"=253, "Blue"=253}, {"Red"=254, "Green"=254, "Blue"=254}, {"Red"=255, "Green"=255, "Blue"=255}] ("Color Palette") cluster{"Red":u8, "Green":u8, "Blue":u8}[] [{"Red"=0, "Green"=0, "Blue"=255}, {"Red"=1, "Green"=1, "Blue"=1}, {"Red"=2, "Green"=2, "Blue"=2}, {"Red"=3, "Green"=3, "Blue"=3}, {"Red"=4, "Green"=4, "Blue"=4}, {"Red"=5, "Green"=5, "Blue"=5}, {"Red"=6, "Green"=6, "Blue"=6}, {"Red"=7, "Green"=7, "Blue"=7}, {"Red"=8, "Green"=8, "Blue"=8}, {"Red"=9, "Green"=9, "Blue"=9}, {"Red"=10, "Green"=10, "Blue"=10}, {"Red"=11, "Green"=11, "Blue"=11}, {"Red"=12, "Green"=12, "Blue"=12}, {"Red"=13, "Green"=13, "Blue"=13}, {"Red"=14, "Green"=14, "Blue"=14}, {"Red"=15, "Green"=15, "Blue"=15}, {"Red"=16, "Green"=16, "Blue"=16}, {"Red"=17, "Green"=17, "Blue"=17}, {"Red"=18, "Green"=18, "Blue"=18}, {"Red"=19, "Green"=19, "Blue"=19}, {"Red"=20, "Green"=20, "Blue"=20}, {"Red"=21, "Green"=21, "Blue"=21}, {"Red"=22, "Green"=22, "Blue"=22}, {"Red"=23, "Green"=23, "Blue"=23}, {"Red"=24, "Green"=24, "Blue"=24}, {"Red"=25, "Green"=25, "Blue"=25}, {"Red"=26, "Green"=26, "Blue"=26}, {"Red"=27, "Green"=27, "Blue"=27}, {"Red"=28, "Green"=28, "Blue"=28}, {"Red"=29, "Green"=29, "Blue"=29}, {"Red"=30, "Green"=30, "Blue"=30}, {"Red"=31, "Green"=31, "Blue"=31}, {"Red"=32, "Green"=32, "Blue"=32}, {"Red"=33, "Green"=33, "Blue"=33}, {"Red"=34, "Green"=34, "Blue"=34}, {"Red"=35, "Green"=35, "Blue"=35}, {"Red"=36, "Green"=36, "Blue"=36}, {"Red"=37, "Green"=37, "Blue"=37}, {"Red"=38, "Green"=38, "Blue"=38}, {"Red"=39, "Green"=39, "Blue"=39}, {"Red"=40, "Green"=40, "Blue"=40}, {"Red"=41, "Green"=41, "Blue"=41}, {"Red"=42, "Green"=42, "Blue"=42}, {"Red"=43, "Green"=43, "Blue"=43}, {"Red"=44, "Green"=44, "Blue"=44}, {"Red"=45, "Green"=45, "Blue"=45}, {"Red"=46, "Green"=46, "Blue"=46}, {"Red"=47, "Green"=47, "Blue"=47}, {"Red"=48, "Green"=48, "Blue"=48}, {"Red"=49, "Green"=49, "Blue"=49}, {"Red"=50, "Green"=50, "Blue"=50}, {"Red"=51, "Green"=51, "Blue"=51}, {"Red"=52, "Green"=52, "Blue"=52}, {"Red"=53, "Green"=53, "Blue"=53}, {"Red"=54, "Green"=54, "Blue"=54}, {"Red"=55, "Green"=55, "Blue"=55}, {"Red"=56, "Green"=56, "Blue"=56}, {"Red"=57, "Green"=57, "Blue"=57}, {"Red"=58, "Green"=58, "Blue"=58}, {"Red"=59, "Green"=59, "Blue"=59}, {"Red"=60, "Green"=60, "Blue"=60}, {"Red"=61, "Green"=61, "Blue"=61}, {"Red"=62, "Green"=62, "Blue"=62}, {"Red"=63, "Green"=63, "Blue"=63}, {"Red"=64, "Green"=64, "Blue"=64}, {"Red"=65, "Green"=65, "Blue"=65}, {"Red"=66, "Green"=66, "Blue"=66}, {"Red"=67, "Green"=67, "Blue"=67}, {"Red"=68, "Green"=68, "Blue"=68}, {"Red"=69, "Green"=69, "Blue"=69}, {"Red"=70, "Green"=70, "Blue"=70}, {"Red"=71, "Green"=71, "Blue"=71}, {"Red"=72, "Green"=72, "Blue"=72}, {"Red"=73, "Green"=73, "Blue"=73}, {"Red"=74, "Green"=74, "Blue"=74}, {"Red"=75, "Green"=75, "Blue"=75}, {"Red"=76, "Green"=76, "Blue"=76}, {"Red"=77, "Green"=77, "Blue"=77}, {"Red"=78, "Green"=78, "Blue"=78}, {"Red"=79, "Green"=79, "Blue"=79}, {"Red"=80, "Green"=80, "Blue"=80}, {"Red"=81, "Green"=81, "Blue"=81}, {"Red"=82, "Green"=82, "Blue"=82}, {"Red"=83, "Green"=83, "Blue"=83}, {"Red"=84, "Green"=84, "Blue"=84}, {"Red"=85, "Green"=85, "Blue"=85}, {"Red"=86, "Green"=86, "Blue"=86}, {"Red"=87, "Green"=87, "Blue"=87}, {"Red"=88, "Green"=88, "Blue"=88}, {"Red"=89, "Green"=89, "Blue"=89}, {"Red"=90, "Green"=90, "Blue"=90}, {"Red"=91, "Green"=91, "Blue"=91}, {"Red"=92, "Green"=92, "Blue"=92}, {"Red"=93, "Green"=93, "Blue"=93}, {"Red"=94, "Green"=94, "Blue"=94}, {"Red"=95, "Green"=95, "Blue"=95}, {"Red"=96, "Green"=96, "Blue"=96}, {"Red"=97, "Green"=97, "Blue"=97}, {"Red"=98, "Green"=98, "Blue"=98}, {"Red"=99, "Green"=99, "Blue"=99}, {"Red"=100, "Green"=100, "Blue"=100}, {"Red"=101, "Green"=101, "Blue"=101}, {"Red"=102, "Green"=102, "Blue"=102}, {"Red"=103, "Green"=103, "Blue"=103}, {"Red"=104, "Green"=104, "Blue"=104}, {"Red"=105, "Green"=105, "Blue"=105}, {"Red"=106, "Green"=106, "Blue"=106}, {"Red"=107, "Green"=107, "Blue"=107}, {"Red"=108, "Green"=108, "Blue"=108}, {"Red"=109, "Green"=109, "Blue"=109}, {"Red"=110, "Green"=110, "Blue"=110}, {"Red"=111, "Green"=111, "Blue"=111}, {"Red"=112, "Green"=112, "Blue"=112}, {"Red"=113, "Green"=113, "Blue"=113}, {"Red"=114, "Green"=114, "Blue"=114}, {"Red"=115, "Green"=115, "Blue"=115}, {"Red"=116, "Green"=116, "Blue"=116}, {"Red"=117, "Green"=117, "Blue"=117}, {"Red"=118, "Green"=118, "Blue"=118}, {"Red"=119, "Green"=119, "Blue"=119}, {"Red"=120, "Green"=120, "Blue"=120}, {"Red"=121, "Green"=121, "Blue"=121}, {"Red"=122, "Green"=122, "Blue"=122}, {"Red"=123, "Green"=123, "Blue"=123}, {"Red"=124, "Green"=124, "Blue"=124}, {"Red"=125, "Green"=125, "Blue"=125}, {"Red"=126, "Green"=126, "Blue"=126}, {"Red"=127, "Green"=127, "Blue"=127}, {"Red"=128, "Green"=128, "Blue"=128}, {"Red"=129, "Green"=129, "Blue"=129}, {"Red"=130, "Green"=130, "Blue"=130}, {"Red"=131, "Green"=131, "Blue"=131}, {"Red"=132, "Green"=132, "Blue"=132}, {"Red"=133, "Green"=133, "Blue"=133}, {"Red"=134, "Green"=134, "Blue"=134}, {"Red"=135, "Green"=135, "Blue"=135}, {"Red"=136, "Green"=136, "Blue"=136}, {"Red"=137, "Green"=137, "Blue"=137}, {"Red"=138, "Green"=138, "Blue"=138}, {"Red"=139, "Green"=139, "Blue"=139}, {"Red"=140, "Green"=140, "Blue"=140}, {"Red"=141, "Green"=141, "Blue"=141}, {"Red"=142, "Green"=142, "Blue"=142}, {"Red"=143, "Green"=143, "Blue"=143}, {"Red"=144, "Green"=144, "Blue"=144}, {"Red"=145, "Green"=145, "Blue"=145}, {"Red"=146, "Green"=146, "Blue"=146}, {"Red"=147, "Green"=147, "Blue"=147}, {"Red"=148, "Green"=148, "Blue"=148}, {"Red"=149, "Green"=149, "Blue"=149}, {"Red"=150, "Green"=150, "Blue"=150}, {"Red"=151, "Green"=151, "Blue"=151}, {"Red"=152, "Green"=152, "Blue"=152}, {"Red"=153, "Green"=153, "Blue"=153}, {"Red"=154, "Green"=154, "Blue"=154}, {"Red"=155, "Green"=155, "Blue"=155}, {"Red"=156, "Green"=156, "Blue"=156}, {"Red"=157, "Green"=157, "Blue"=157}, {"Red"=158, "Green"=158, "Blue"=158}, {"Red"=159, "Green"=159, "Blue"=159}, {"Red"=160, "Green"=160, "Blue"=160}, {"Red"=161, "Green"=161, "Blue"=161}, {"Red"=162, "Green"=162, "Blue"=162}, {"Red"=163, "Green"=163, "Blue"=163}, {"Red"=164, "Green"=164, "Blue"=164}, {"Red"=165, "Green"=165, "Blue"=165}, {"Red"=166, "Green"=166, "Blue"=166}, {"Red"=167, "Green"=167, "Blue"=167}, {"Red"=168, "Green"=168, "Blue"=168}, {"Red"=169, "Green"=169, "Blue"=169}, {"Red"=170, "Green"=170, "Blue"=170}, {"Red"=171, "Green"=171, "Blue"=171}, {"Red"=172, "Green"=172, "Blue"=172}, {"Red"=173, "Green"=173, "Blue"=173}, {"Red"=174, "Green"=174, "Blue"=174}, {"Red"=175, "Green"=175, "Blue"=175}, {"Red"=176, "Green"=176, "Blue"=176}, {"Red"=177, "Green"=177, "Blue"=177}, {"Red"=178, "Green"=178, "Blue"=178}, {"Red"=179, "Green"=179, "Blue"=179}, {"Red"=180, "Green"=180, "Blue"=180}, {"Red"=181, "Green"=181, "Blue"=181}, {"Red"=182, "Green"=182, "Blue"=182}, {"Red"=183, "Green"=183, "Blue"=183}, {"Red"=184, "Green"=184, "Blue"=184}, {"Red"=185, "Green"=185, "Blue"=185}, {"Red"=186, "Green"=186, "Blue"=186}, {"Red"=187, "Green"=187, "Blue"=187}, {"Red"=188, "Green"=188, "Blue"=188}, {"Red"=189, "Green"=189, "Blue"=189}, {"Red"=190, "Green"=190, "Blue"=190}, {"Red"=191, "Green"=191, "Blue"=191}, {"Red"=192, "Green"=192, "Blue"=192}, {"Red"=193, "Green"=193, "Blue"=193}, {"Red"=194, "Green"=194, "Blue"=194}, {"Red"=195, "Green"=195, "Blue"=195}, {"Red"=196, "Green"=196, "Blue"=196}, {"Red"=197, "Green"=197, "Blue"=197}, {"Red"=198, "Green"=198, "Blue"=198}, {"Red"=199, "Green"=199, "Blue"=199}, {"Red"=200, "Green"=200, "Blue"=200}, {"Red"=201, "Green"=201, "Blue"=201}, {"Red"=202, "Green"=202, "Blue"=202}, {"Red"=203, "Green"=203, "Blue"=203}, {"Red"=204, "Green"=204, "Blue"=204}, {"Red"=205, "Green"=205, "Blue"=205}, {"Red"=206, "Green"=206, "Blue"=206}, {"Red"=207, "Green"=207, "Blue"=207}, {"Red"=208, "Green"=208, "Blue"=208}, {"Red"=209, "Green"=209, "Blue"=209}, {"Red"=210, "Green"=210, "Blue"=210}, {"Red"=211, "Green"=211, "Blue"=211}, {"Red"=212, "Green"=212, "Blue"=212}, {"Red"=213, "Green"=213, "Blue"=213}, {"Red"=214, "Green"=214, "Blue"=214}, {"Red"=215, "Green"=215, "Blue"=215}, {"Red"=216, "Green"=216, "Blue"=216}, {"Red"=217, "Green"=217, "Blue"=217}, {"Red"=218, "Green"=218, "Blue"=218}, {"Red"=219, "Green"=219, "Blue"=219}, {"Red"=220, "Green"=220, "Blue"=220}, {"Red"=221, "Green"=221, "Blue"=221}, {"Red"=222, "Green"=222, "Blue"=222}, {"Red"=223, "Green"=223, "Blue"=223}, {"Red"=224, "Green"=224, "Blue"=224}, {"Red"=225, "Green"=225, "Blue"=225}, {"Red"=226, "Green"=226, "Blue"=226}, {"Red"=227, "Green"=227, "Blue"=227}, {"Red"=228, "Green"=228, "Blue"=228}, {"Red"=229, "Green"=229, "Blue"=229}, {"Red"=230, "Green"=230, "Blue"=230}, {"Red"=231, "Green"=231, "Blue"=231}, {"Red"=232, "Green"=232, "Blue"=232}, {"Red"=233, "Green"=233, "Blue"=233}, {"Red"=234, "Green"=234, "Blue"=234}, {"Red"=235, "Green"=235, "Blue"=235}, {"Red"=236, "Green"=236, "Blue"=236}, {"Red"=237, "Green"=237, "Blue"=237}, {"Red"=238, "Green"=238, "Blue"=238}, {"Red"=239, "Green"=239, "Blue"=239}, {"Red"=240, "Green"=240, "Blue"=240}, {"Red"=241, "Green"=241, "Blue"=241}, {"Red"=242, "Green"=242, "Blue"=242}, {"Red"=243, "Green"=243, "Blue"=243}, {"Red"=244, "Green"=244, "Blue"=244}, {"Red"=245, "Green"=245, "Blue"=245}, {"Red"=246, "Green"=246, "Blue"=246}, {"Red"=247, "Green"=247, "Blue"=247}, {"Red"=248, "Green"=248, "Blue"=248}, {"Red"=249, "Green"=249, "Blue"=249}, {"Red"=250, "Green"=250, "Blue"=250}, {"Red"=251, "Green"=251, "Blue"=251}, {"Red"=252, "Green"=252, "Blue"=252}, {"Red"=253, "Green"=253, "Blue"=253}, {"Red"=254, "Green"=254, "Blue"=254}, {"Red"=255, "Green"=0, "Blue"=0}] ("Color Palette") cluster{"Red":u8, "Green":u8, "Blue":u8}[] [{"Red"=0, "Green"=0, "Blue"=0}, {"Red"=1, "Green"=1, "Blue"=1}, {"Red"=2, "Green"=2, "Blue"=2}, {"Red"=3, "Green"=3, "Blue"=3}, {"Red"=4, "Green"=4, "Blue"=4}, {"Red"=5, "Green"=5, "Blue"=5}, {"Red"=6, "Green"=6, "Blue"=6}, {"Red"=7, "Green"=7, "Blue"=7}, {"Red"=8, "Green"=8, "Blue"=8}, {"Red"=9, "Green"=9, "Blue"=9}, {"Red"=10, "Green"=10, "Blue"=10}, {"Red"=11, "Green"=11, "Blue"=11}, {"Red"=12, "Green"=12, "Blue"=12}, {"Red"=13, "Green"=13, "Blue"=13}, {"Red"=14, "Green"=14, "Blue"=14}, {"Red"=15, "Green"=15, "Blue"=15}, {"Red"=16, "Green"=16, "Blue"=16}, {"Red"=17, "Green"=17, "Blue"=17}, {"Red"=18, "Green"=18, "Blue"=18}, {"Red"=19, "Green"=19, "Blue"=19}, {"Red"=20, "Green"=20, "Blue"=20}, {"Red"=21, "Green"=21, "Blue"=21}, {"Red"=22, "Green"=22, "Blue"=22}, {"Red"=23, "Green"=23, "Blue"=23}, {"Red"=24, "Green"=24, "Blue"=24}, {"Red"=25, "Green"=25, "Blue"=25}, {"Red"=26, "Green"=26, "Blue"=26}, {"Red"=27, "Green"=27, "Blue"=27}, {"Red"=28, "Green"=28, "Blue"=28}, {"Red"=29, "Green"=29, "Blue"=29}, {"Red"=30, "Green"=30, "Blue"=30}, {"Red"=31, "Green"=31, "Blue"=31}, {"Red"=32, "Green"=32, "Blue"=32}, {"Red"=33, "Green"=33, "Blue"=33}, {"Red"=34, "Green"=34, "Blue"=34}, {"Red"=35, "Green"=35, "Blue"=35}, {"Red"=36, "Green"=36, "Blue"=36}, {"Red"=37, "Green"=37, "Blue"=37}, {"Red"=38, "Green"=38, "Blue"=38}, {"Red"=39, "Green"=39, "Blue"=39}, {"Red"=40, "Green"=40, "Blue"=40}, {"Red"=41, "Green"=41, "Blue"=41}, {"Red"=42, "Green"=42, "Blue"=42}, {"Red"=43, "Green"=43, "Blue"=43}, {"Red"=44, "Green"=44, "Blue"=44}, {"Red"=45, "Green"=45, "Blue"=45}, {"Red"=46, "Green"=46, "Blue"=46}, {"Red"=47, "Green"=47, "Blue"=47}, {"Red"=48, "Green"=48, "Blue"=48}, {"Red"=49, "Green"=49, "Blue"=49}, {"Red"=50, "Green"=50, "Blue"=50}, {"Red"=51, "Green"=51, "Blue"=51}, {"Red"=52, "Green"=52, "Blue"=52}, {"Red"=53, "Green"=53, "Blue"=53}, {"Red"=54, "Green"=54, "Blue"=54}, {"Red"=55, "Green"=55, "Blue"=55}, {"Red"=56, "Green"=56, "Blue"=56}, {"Red"=57, "Green"=57, "Blue"=57}, {"Red"=58, "Green"=58, "Blue"=58}, {"Red"=59, "Green"=59, "Blue"=59}, {"Red"=60, "Green"=60, "Blue"=60}, {"Red"=61, "Green"=61, "Blue"=61}, {"Red"=62, "Green"=62, "Blue"=62}, {"Red"=63, "Green"=63, "Blue"=63}, {"Red"=64, "Green"=64, "Blue"=64}, {"Red"=65, "Green"=65, "Blue"=65}, {"Red"=66, "Green"=66, "Blue"=66}, {"Red"=67, "Green"=67, "Blue"=67}, {"Red"=68, "Green"=68, "Blue"=68}, {"Red"=69, "Green"=69, "Blue"=69}, {"Red"=70, "Green"=70, "Blue"=70}, {"Red"=71, "Green"=71, "Blue"=71}, {"Red"=72, "Green"=72, "Blue"=72}, {"Red"=73, "Green"=73, "Blue"=73}, {"Red"=74, "Green"=74, "Blue"=74}, {"Red"=75, "Green"=75, "Blue"=75}, {"Red"=76, "Green"=76, "Blue"=76}, {"Red"=77, "Green"=77, "Blue"=77}, {"Red"=78, "Green"=78, "Blue"=78}, {"Red"=79, "Green"=79, "Blue"=79}, {"Red"=80, "Green"=80, "Blue"=80}, {"Red"=81, "Green"=81, "Blue"=81}, {"Red"=82, "Green"=82, "Blue"=82}, {"Red"=83, "Green"=83, "Blue"=83}, {"Red"=84, "Green"=84, "Blue"=84}, {"Red"=85, "Green"=85, "Blue"=85}, {"Red"=86, "Green"=86, "Blue"=86}, {"Red"=87, "Green"=87, "Blue"=87}, {"Red"=88, "Green"=88, "Blue"=88}, {"Red"=89, "Green"=89, "Blue"=89}, {"Red"=90, "Green"=90, "Blue"=90}, {"Red"=91, "Green"=91, "Blue"=91}, {"Red"=92, "Green"=92, "Blue"=92}, {"Red"=93, "Green"=93, "Blue"=93}, {"Red"=94, "Green"=94, "Blue"=94}, {"Red"=95, "Green"=95, "Blue"=95}, {"Red"=96, "Green"=96, "Blue"=96}, {"Red"=97, "Green"=97, "Blue"=97}, {"Red"=98, "Green"=98, "Blue"=98}, {"Red"=99, "Green"=99, "Blue"=99}, {"Red"=100, "Green"=100, "Blue"=100}, {"Red"=101, "Green"=101, "Blue"=101}, {"Red"=102, "Green"=102, "Blue"=102}, {"Red"=103, "Green"=103, "Blue"=103}, {"Red"=104, "Green"=104, "Blue"=104}, {"Red"=105, "Green"=105, "Blue"=105}, {"Red"=106, "Green"=106, "Blue"=106}, {"Red"=107, "Green"=107, "Blue"=107}, {"Red"=108, "Green"=108, "Blue"=108}, {"Red"=109, "Green"=109, "Blue"=109}, {"Red"=110, "Green"=110, "Blue"=110}, {"Red"=111, "Green"=111, "Blue"=111}, {"Red"=112, "Green"=112, "Blue"=112}, {"Red"=113, "Green"=113, "Blue"=113}, {"Red"=114, "Green"=114, "Blue"=114}, {"Red"=115, "Green"=115, "Blue"=115}, {"Red"=116, "Green"=116, "Blue"=116}, {"Red"=117, "Green"=117, "Blue"=117}, {"Red"=118, "Green"=118, "Blue"=118}, {"Red"=119, "Green"=119, "Blue"=119}, {"Red"=120, "Green"=120, "Blue"=120}, {"Red"=121, "Green"=121, "Blue"=121}, {"Red"=122, "Green"=122, "Blue"=122}, {"Red"=123, "Green"=123, "Blue"=123}, {"Red"=124, "Green"=124, "Blue"=124}, {"Red"=125, "Green"=125, "Blue"=125}, {"Red"=126, "Green"=126, "Blue"=126}, {"Red"=127, "Green"=127, "Blue"=127}, {"Red"=128, "Green"=128, "Blue"=128}, {"Red"=129, "Green"=129, "Blue"=129}, {"Red"=130, "Green"=130, "Blue"=130}, {"Red"=131, "Green"=131, "Blue"=131}, {"Red"=132, "Green"=132, "Blue"=132}, {"Red"=133, "Green"=133, "Blue"=133}, {"Red"=134, "Green"=134, "Blue"=134}, {"Red"=135, "Green"=135, "Blue"=135}, {"Red"=136, "Green"=136, "Blue"=136}, {"Red"=137, "Green"=137, "Blue"=137}, {"Red"=138, "Green"=138, "Blue"=138}, {"Red"=139, "Green"=139, "Blue"=139}, {"Red"=140, "Green"=140, "Blue"=140}, {"Red"=141, "Green"=141, "Blue"=141}, {"Red"=142, "Green"=142, "Blue"=142}, {"Red"=143, "Green"=143, "Blue"=143}, {"Red"=144, "Green"=144, "Blue"=144}, {"Red"=145, "Green"=145, "Blue"=145}, {"Red"=146, "Green"=146, "Blue"=146}, {"Red"=147, "Green"=147, "Blue"=147}, {"Red"=148, "Green"=148, "Blue"=148}, {"Red"=149, "Green"=149, "Blue"=149}, {"Red"=150, "Green"=150, "Blue"=150}, {"Red"=151, "Green"=151, "Blue"=151}, {"Red"=152, "Green"=152, "Blue"=152}, {"Red"=153, "Green"=153, "Blue"=153}, {"Red"=154, "Green"=154, "Blue"=154}, {"Red"=155, "Green"=155, "Blue"=155}, {"Red"=156, "Green"=156, "Blue"=156}, {"Red"=157, "Green"=157, "Blue"=157}, {"Red"=158, "Green"=158, "Blue"=158}, {"Red"=159, "Green"=159, "Blue"=159}, {"Red"=160, "Green"=160, "Blue"=160}, {"Red"=161, "Green"=161, "Blue"=161}, {"Red"=162, "Green"=162, "Blue"=162}, {"Red"=163, "Green"=163, "Blue"=163}, {"Red"=164, "Green"=164, "Blue"=164}, {"Red"=165, "Green"=165, "Blue"=165}, {"Red"=166, "Green"=166, "Blue"=166}, {"Red"=167, "Green"=167, "Blue"=167}, {"Red"=168, "Green"=168, "Blue"=168}, {"Red"=169, "Green"=169, "Blue"=169}, {"Red"=170, "Green"=170, "Blue"=170}, {"Red"=171, "Green"=171, "Blue"=171}, {"Red"=172, "Green"=172, "Blue"=172}, {"Red"=173, "Green"=173, "Blue"=173}, {"Red"=174, "Green"=174, "Blue"=174}, {"Red"=175, "Green"=175, "Blue"=175}, {"Red"=176, "Green"=176, "Blue"=176}, {"Red"=177, "Green"=177, "Blue"=177}, {"Red"=178, "Green"=178, "Blue"=178}, {"Red"=179, "Green"=179, "Blue"=179}, {"Red"=180, "Green"=180, "Blue"=180}, {"Red"=181, "Green"=181, "Blue"=181}, {"Red"=182, "Green"=182, "Blue"=182}, {"Red"=183, "Green"=183, "Blue"=183}, {"Red"=184, "Green"=184, "Blue"=184}, {"Red"=185, "Green"=185, "Blue"=185}, {"Red"=186, "Green"=186, "Blue"=186}, {"Red"=187, "Green"=187, "Blue"=187}, {"Red"=188, "Green"=188, "Blue"=188}, {"Red"=189, "Green"=189, "Blue"=189}, {"Red"=190, "Green"=190, "Blue"=190}, {"Red"=191, "Green"=191, "Blue"=191}, {"Red"=192, "Green"=192, "Blue"=192}, {"Red"=193, "Green"=193, "Blue"=193}, {"Red"=194, "Green"=194, "Blue"=194}, {"Red"=195, "Green"=195, "Blue"=195}, {"Red"=196, "Green"=196, "Blue"=196}, {"Red"=197, "Green"=197, "Blue"=197}, {"Red"=198, "Green"=198, "Blue"=198}, {"Red"=199, "Green"=199, "Blue"=199}, {"Red"=200, "Green"=200, "Blue"=200}, {"Red"=201, "Green"=201, "Blue"=201}, {"Red"=202, "Green"=202, "Blue"=202}, {"Red"=203, "Green"=203, "Blue"=203}, {"Red"=204, "Green"=204, "Blue"=204}, {"Red"=205, "Green"=205, "Blue"=205}, {"Red"=206, "Green"=206, "Blue"=206}, {"Red"=207, "Green"=207, "Blue"=207}, {"Red"=208, "Green"=208, "Blue"=208}, {"Red"=209, "Green"=209, "Blue"=209}, {"Red"=210, "Green"=210, "Blue"=210}, {"Red"=211, "Green"=211, "Blue"=211}, {"Red"=212, "Green"=212, "Blue"=212}, {"Red"=213, "Green"=213, "Blue"=213}, {"Red"=214, "Green"=214, "Blue"=214}, {"Red"=215, "Green"=215, "Blue"=215}, {"Red"=216, "Green"=216, "Blue"=216}, {"Red"=217, "Green"=217, "Blue"=217}, {"Red"=218, "Green"=218, "Blue"=218}, {"Red"=219, "Green"=219, "Blue"=219}, {"Red"=220, "Green"=220, "Blue"=220}, {"Red"=221, "Green"=221, "Blue"=221}, {"Red"=222, "Green"=222, "Blue"=222}, {"Red"=223, "Green"=223, "Blue"=223}, {"Red"=224, "Green"=224, "Blue"=224}, {"Red"=225, "Green"=225, "Blue"=225}, {"Red"=226, "Green"=226, "Blue"=226}, {"Red"=227, "Green"=227, "Blue"=227}, {"Red"=228, "Green"=228, "Blue"=228}, {"Red"=229, "Green"=229, "Blue"=229}, {"Red"=230, "Green"=230, "Blue"=230}, {"Red"=231, "Green"=231, "Blue"=231}, {"Red"=232, "Green"=232, "Blue"=232}, {"Red"=233, "Green"=233, "Blue"=233}, {"Red"=234, "Green"=234, "Blue"=234}, {"Red"=235, "Green"=235, "Blue"=235}, {"Red"=236, "Green"=236, "Blue"=236}, {"Red"=237, "Green"=237, "Blue"=237}, {"Red"=238, "Green"=238, "Blue"=238}, {"Red"=239, "Green"=239, "Blue"=239}, {"Red"=240, "Green"=240, "Blue"=240}, {"Red"=241, "Green"=241, "Blue"=241}, {"Red"=242, "Green"=242, "Blue"=242}, {"Red"=243, "Green"=243, "Blue"=243}, {"Red"=244, "Green"=244, "Blue"=244}, {"Red"=245, "Green"=245, "Blue"=245}, {"Red"=246, "Green"=246, "Blue"=246}, {"Red"=247, "Green"=247, "Blue"=247}, {"Red"=248, "Green"=248, "Blue"=248}, {"Red"=249, "Green"=249, "Blue"=249}, {"Red"=250, "Green"=250, "Blue"=250}, {"Red"=251, "Green"=251, "Blue"=251}, {"Red"=252, "Green"=252, "Blue"=252}, {"Red"=253, "Green"=253, "Blue"=253}, {"Red"=254, "Green"=254, "Blue"=254}, {"Red"=255, "Green"=255, "Blue"=255}] ("Color Palette")] -> w51
            frame "high clipping red" {
            }
            frame "low clipping blue" {
            }
            frame "high and low clipping" {
            }
            frame "standard", "high / low (full range)" {
            }
          }
          n51 = case shown="\"Reso\"" w40 {
            tunnel: w39 -> [w72 w77]
            tunnel: w38 -> [w71 w76]
            tunnel: [w72 w73] -> w37
            tunnel: [w71 w74] -> w36
            frame "Galvo", Default {
            }
            frame "Reso" {
              w75 = 32767  # offset
              n52 = Subtract(x=w77, y=w75) -> (x-y=w73:i32)
              n53 = Subtract(x=w76, y=w75) -> (x-y=w74:i32)
            }
          }
          n54 = property class="ImageControl"(reference=w46, error in=w60, "16-bit Display Conversion Method"=w63, "16-bit Display Maximum Value"=w36, "Palette Type"=w52, "User Palette"=w51) -> (reference out=w50:refnum<vi>, error out=w49:errorcluster)
          n55 = property class="ImageControl"(reference=w50, error in=w49, "16-bit Display Minimum Value"=w37) -> (reference out=w48:refnum<vi>, error out=w47:errorcluster)
        }
      }
      n56 = Close Reference(reference=w29, error in (no error)=w28) -> (error out=w22:errorcluster)
    }
    frame Error {
      w179 = i16 -1
    }
  }
  "Error Out" <- w5
  "SciScan Image Tab Number" <- w3
  "Current Image" <- w4
  "Channel Number" <- w2
  "Channel type" <- w1
